vi "DTACQ - Read AWG Length.vi"(8 "error in":errorcluster, 11 "Address":string) -> (0 "error out":errorcluster, 2 "AWG Length":i32)   [LabVIEW 2017, in "Communications Library.lvlib"]
doc: "Querries the status of the DTACQ device.\n\nThe status of both the module carrier and the analog out module are querried."
uses:
  Communications Library.lvlib
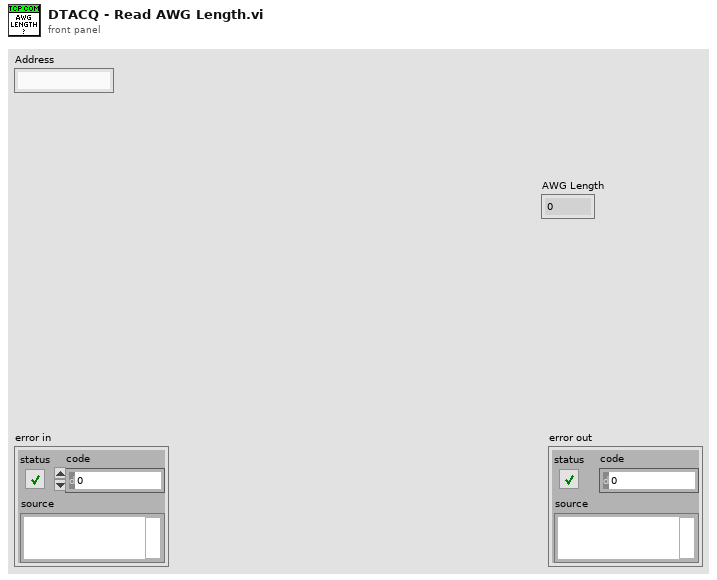
[diagram p1: front panel]
types:
  T1 = typedef "Communications Library.lvlib/DTACQ Connection Data--Cluster.ctl" = cluster{"Description":string, "Address":string, "Port":u16, "timeout (ms)":i32, "Termination Character":string, "TCP Connection Reference":refnum<k5>, "Open Connection":bool}
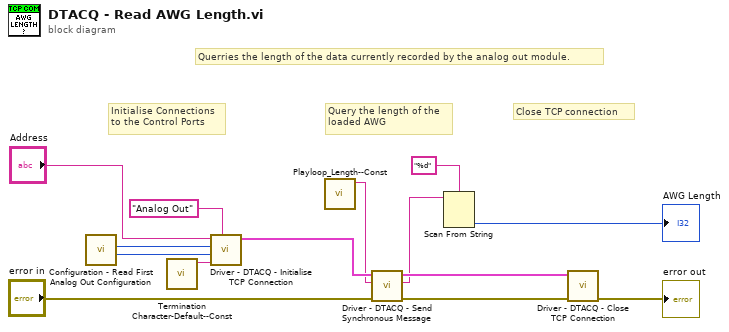
[diagram p0: block diagram]
diagram:
  # "Querries the length of the data currently recorded by the analog out module."
  # "Close TCP connection"
  # "Query the length of the\nloaded AWG"
  # "Initialise Connections\nto the Control Ports"
  n1 = call "Configuration - Read First Analog Out Configuration.vi"() -> ("Timeout (ms)"=w5:i32, "Analog Out Control Port"=w6:i32)  [unwired: 7 in, 3 out]
  n2 = call "Termination Character-Default--Const.vi"() -> ("Termination Character"=w10:string)  [unwired: 11 in]
  n3 = call "Driver - DTACQ - Initialise TCP Connection.vi"("Description"="Analog Out", "Termination Character"=w10, "timeout (ms)"=w5, "Port"=w6, "Address"="Address") -> ("DTACQ Connection Data Out"=w8:T1)  [unwired: 6 in]
  n4 = call "Playloop_Length--Const.vi"() -> ("AWG Length Command"=w4:string)  [unwired: 11 in]
  n5 = call "Driver - DTACQ - Send Synchronous Message.vi"("error in"="error in", "Message to Send"=w4, "DTACQ Connection Data In"=w8) -> ("error out"=w12:errorcluster, "Read String"=w3:string, "DTACQ Connection Data Out"=w13:T1)  [unwired: 5 in, 1 out]
  n6 = Scan From String(format string="%d", input string=w3) -> (output 1=→"AWG Length":i32)  [unwired: 3 in, 3 out]
  n7 = call "Driver - DTACQ - Close TCP Connection.vi"("error in"=w12, "DTACQ Connection Data In"=w13) -> ("error out"=→"error out":errorcluster)  [unwired: 8 in, 1 out]
